vi "Save.vi"(8 "error in (no error)":errorcluster, 11 "Data File":path) -> (0 "error out":errorcluster, 3 "dup Data File":path)   [LabVIEW 2014, in "Contact Data.lvlib"]
doc: "Saves the contents of the address book data store to a file on disk that can be used to load the data store again later."
uses:
  Contact Data.lvlib
  Command.ctl
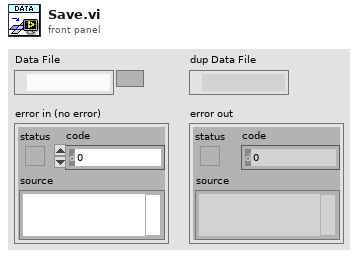
[diagram p1: front panel]
types:
  T1 = typedef "Contact Data.lvlib/Command.ctl" = enum16{"Set All Contacts", "Load", "Save", "Get All Data", "Get Single Data (ID)", "Get Single Data", "Set Position", "Set Destinations", "Set Controls", "Remove Single Data", "Remove UUID Contact", "Set Single ALL", "Is Data Modified", "Import Data"}
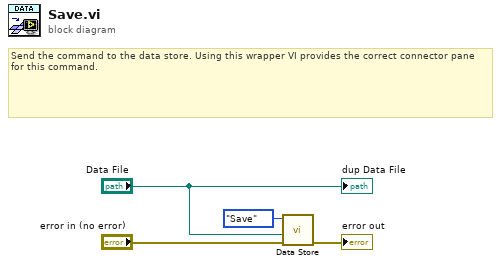
[diagram p0: block diagram]
diagram:
  # "Send the command to the data store. Using this wrapper VI provides the correct connector pane for this command."
  n1 = call "Data Store.vi"("error in (no error)"="error in (no error)", "Data File"="Data File", "Command"=Command."Save") -> ("error out"=→"error out":errorcluster)  [unwired: 6 in, 2 out]
  "dup Data File" <- "Data File"
